vi "Find Attribute.vi"(10 "Name":string, 11 "Attributes":refnum<class "Attribute.lvclass">[](array[class])) -> (1 "Found?":bool, 2 "Value":refnum<class "Data Item.lvclass">, 3 "Attribute":refnum<class "Attribute.lvclass">)   [LabVIEW 2018, in "VILab.lvlib" / "Attribute.lvclass"]
uses:
  Attribute.lvclass
  Data Item.lvclass
  Attribute.lvclass/Attribute.ctl
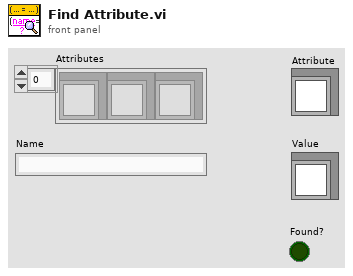
[diagram p1: front panel]
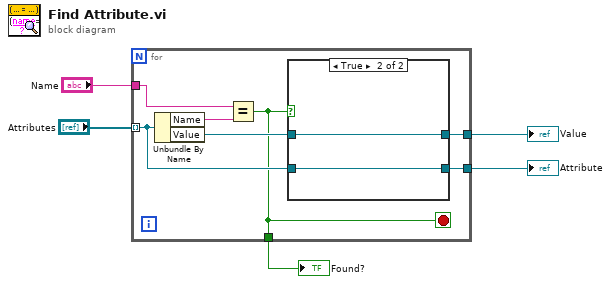
[diagram p0: block diagram]
diagram:
  n1 = for {
    tunnel: "Attributes" -> [w10] mode=indexing
    tunnel: "Name" -> [w11]
    tunnel: [w8] -> w2
    tunnel: [w7] -> w1
    tunnel: [w6] -> w3
    stop <- w6 stop-if-true
    n2 = Unbundle By Name(w10) -> ("Name"=w12:string, "Value"=w9:refnum<class "Data Item.lvclass">)
    n3 = Equal?(x=w11, y=w12) -> (x = y?=w6:bool)
    n4 = case shown="True" w6 {
      tunnel: w10 -> [_ w13]
      tunnel: w9 -> [_ w14]
      tunnel: [_ w14] -> w8
      tunnel: [_ w13] -> w7
      frame False {
      }
      frame True {
      }
    }
  }
  "Value" <- w2
  "Found?" <- w3
  "Attribute" <- w1
